vi "ReadContTrackerResponse.vi"(8 "error in (no error)":errorcluster, 10 "Command":string, 11 "TCP Network Connection in":refnum<k5>) -> (0 "error out":errorcluster, 2 "Respond":string[](array[string]), 3 "TCP Network Connection out":refnum<k5>)   [LabVIEW 2017]
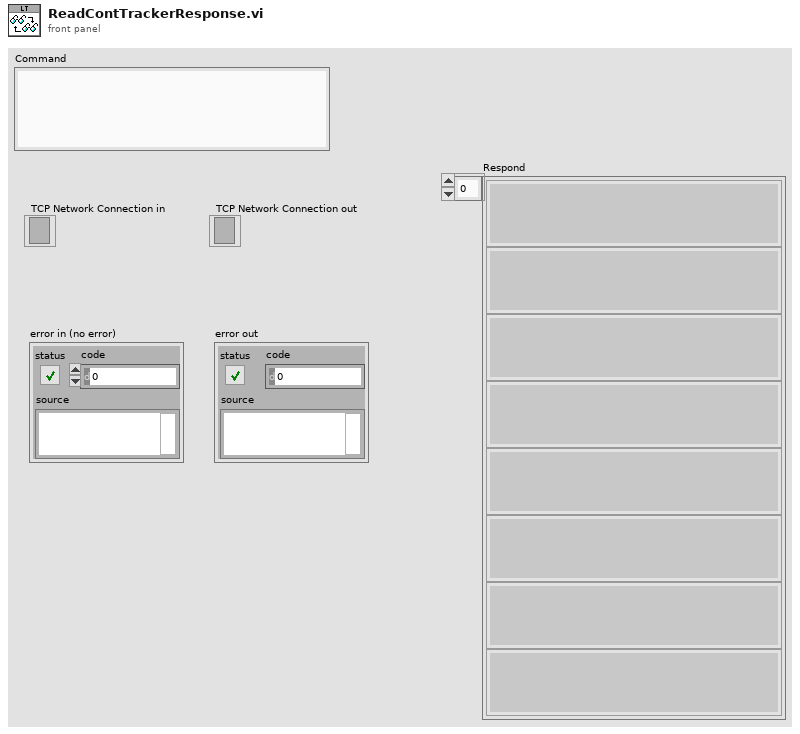
[diagram p1: front panel]
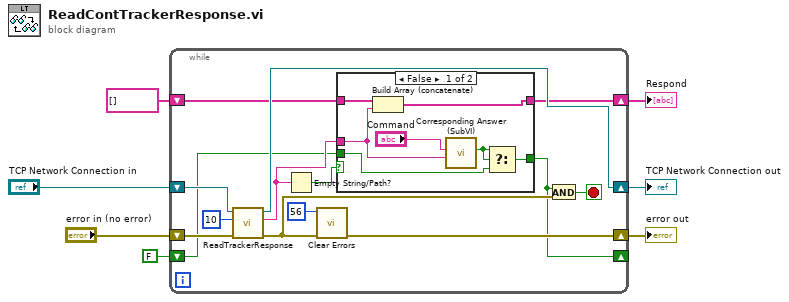
[diagram p0: block diagram]
diagram:
  n1 = while {
    shift-right: [w20] -> w2
    shift-left: "TCP Network Connection in" -> [w21]
    shift-right: [w15] -> w4
    shift-left: "error in (no error)" -> [w19]
    shift-right: [w11] -> w5
    shift-left: string[] [] -> [w10]
    shift-right: [w8] -> _
    shift-left: FALSE ("logical AND") -> [w9]
    stop <- w17 stop-if-true
    n2 = call "ReadTrackerResponse.vi"("error in"=w19, "timeout ms (1000)"=10, "connection ID in"=w21) -> ("error out"=w16:errorcluster, "Tracker Response"=w12:string, "connection ID out"=w20:refnum<k5>)  [unwired: 6 in]
    n3 = Empty String/Path?(string/path=w12) -> (empty?=w13:bool)
    n4 = call <vilib>:"Clear Errors.vi"("error in (no error)"=w16, "specific error code to clear (0: all)"=56) -> ("error out"=w15:errorcluster)  [unwired: 4 in, 1 out]
    n5 = case shown="False" w13 {
      tunnel: w12 -> [w23 _]
      tunnel: [w28 w30] -> w11
      tunnel: w10 -> [w27 w30]
      tunnel: w9 -> [w26 w29]
      tunnel: [w25 w29] -> w8
      frame False {
        n6 = Build Array (concatenate)(w27, w23) -> (w28:string[])
        n7 = call "Corresponding Answer (SubVI).vi"("Command"="Command", "Tracker Response"=w23) -> ("Boolean"=w24:bool)  [unwired: 8 in]
        n8 = Select(t=w24, s=w24, f=w26) -> (s? t:f=w25:bool)
      }
      frame True {
      }
    }
    n9 = And(x=w8, y=w16) -> (x .and. y?=w17:bool)
  }
  "Respond" <- w5
  "error out" <- w4
  "TCP Network Connection out" <- w2
